vi "ADC Data capture and Process.vi"(0 "ADC Output Read Method":T2(ring)=enum."Read .dat file", 1 "Select the Tab to project":T1(ring)=enum."ADC Sine", 2 "ADC Input":enum16{"Sine Wave", "Ramp / Triangle"}(ring), 3 "No.of samples(SNR)":i32=4096, 4 "Resolution":i32=12, 5 "active edge":i32(ring)=10280, 6 "Inputs for Dyanmic para":T9={"Fundamental Frequency"=100000.0, "Sampling Frequncy"=3999610.0, "No of Harmonics"=9, "Window"=enum."7 Term B-Harris", "Blackman (fundamental power) bins)"=1.0}, 7 "Samples per Channel":i32=4096 caption="No.of Samples(capture)", 8 "Oversampling":bool, 9 "Oversampling ratio":i32, 10 "Drop LSB":bool, 11 "Save data":T15, 12 "Waveform":i64[](array[numeric]), 13 "Path to Read":path=path "C/Users/a0230227/Desktop/save.dat", 14 "Start & Stop Bit":cluster{"Start":i32, "Stop":i32}={"Start"=40, "Stop"=4055}, 15 "length":i32=4096, 24 "path to save":T14={"Path to Save plot"=path "D/Tenor_176P/DYN_PAR_C004/DAT/D001_TEMPP30C_VDD1.2_VDDA3.3_16B_SE_ADCA__vicA_aggX_PLT_CAP_200821_1740_33.jpg", "Path to Raw Data plot"=path "D/Tenor_176P/DYN_PAR_C004/DAT/D001_TEMPP30C_VDD1.2_VDDA3.3_16B_SE_ADCA__vicA_aggX_RAW_DAT_200821_1740_33.csv"}) -> (18 "Min Max":T4, 19 "detected Throughput":dbl, 20 "output cluster":T7, 21 "Dynamic Parameters":T8, 22 "max code":ext, 23 "min code":ext, 25 "Valid Capture":bool)   [LabVIEW 2021] (continued)
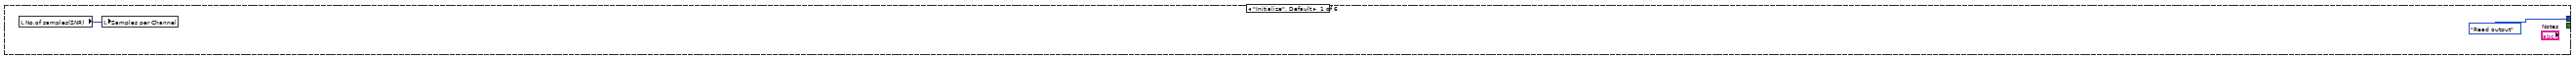
[diagram p2: hidden frame]
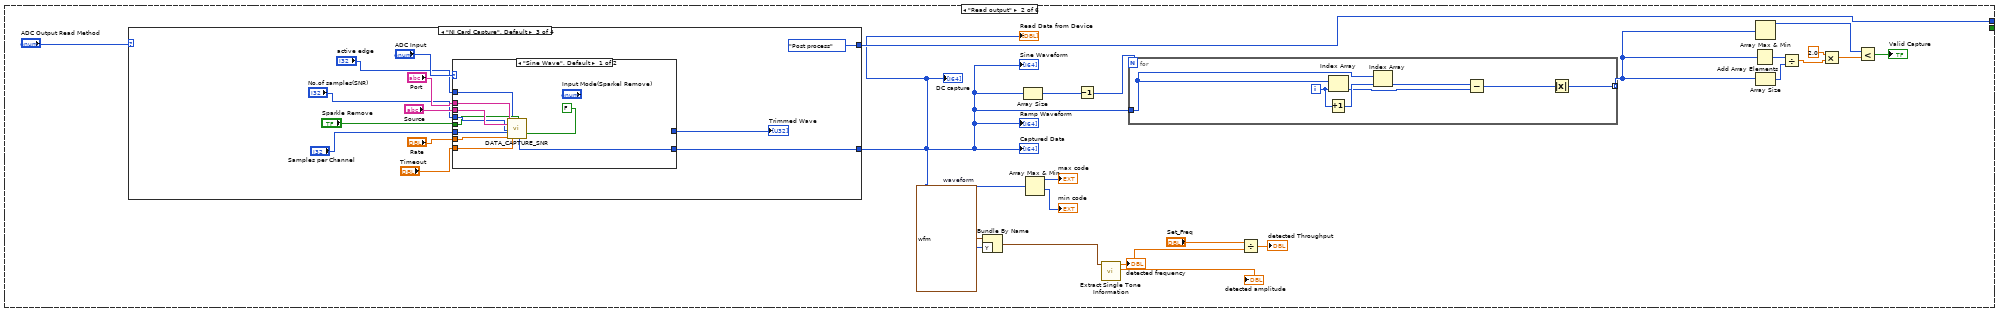
[diagram p3: hidden frame]
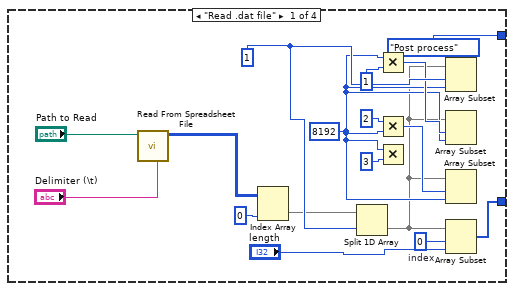
[diagram p4: hidden frame]
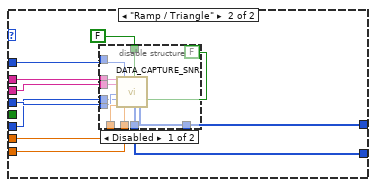
[diagram p6: hidden frame]
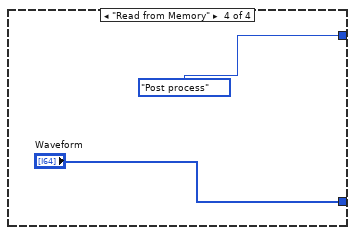
[diagram p8: hidden frame]
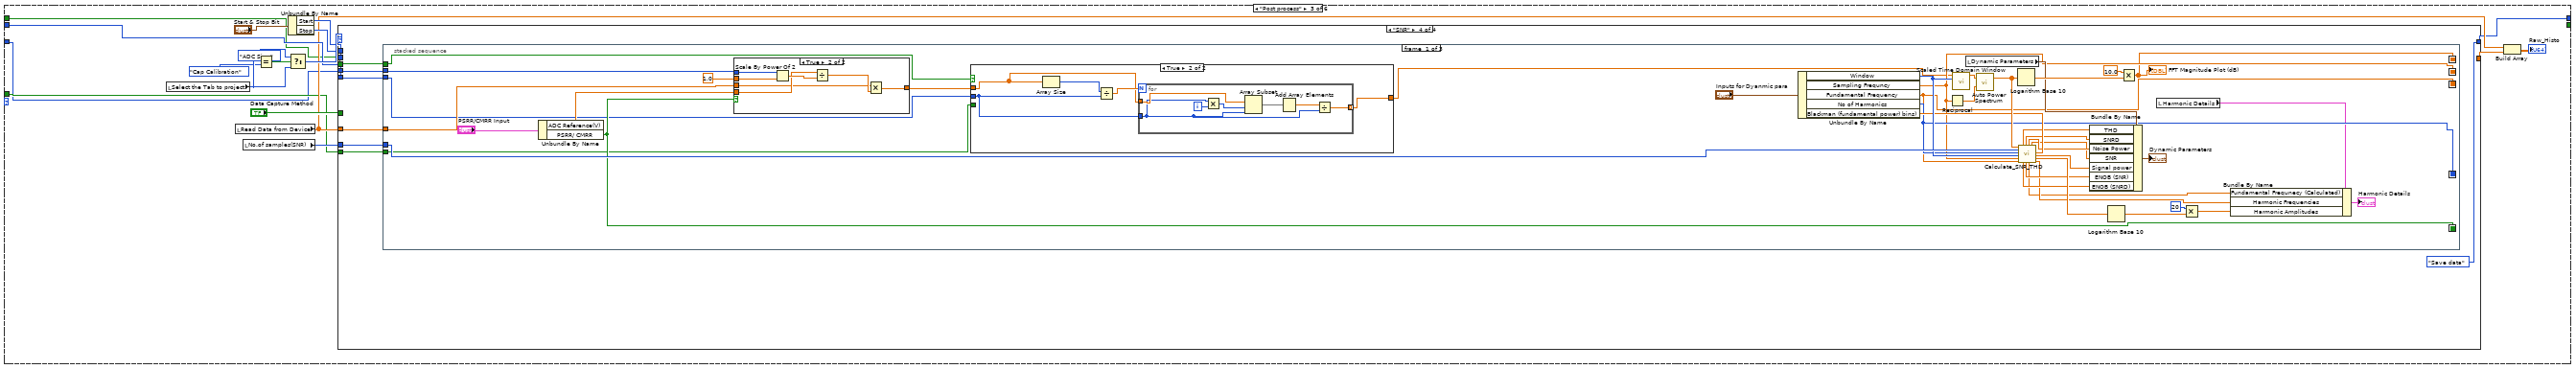
[diagram p9: hidden frame]
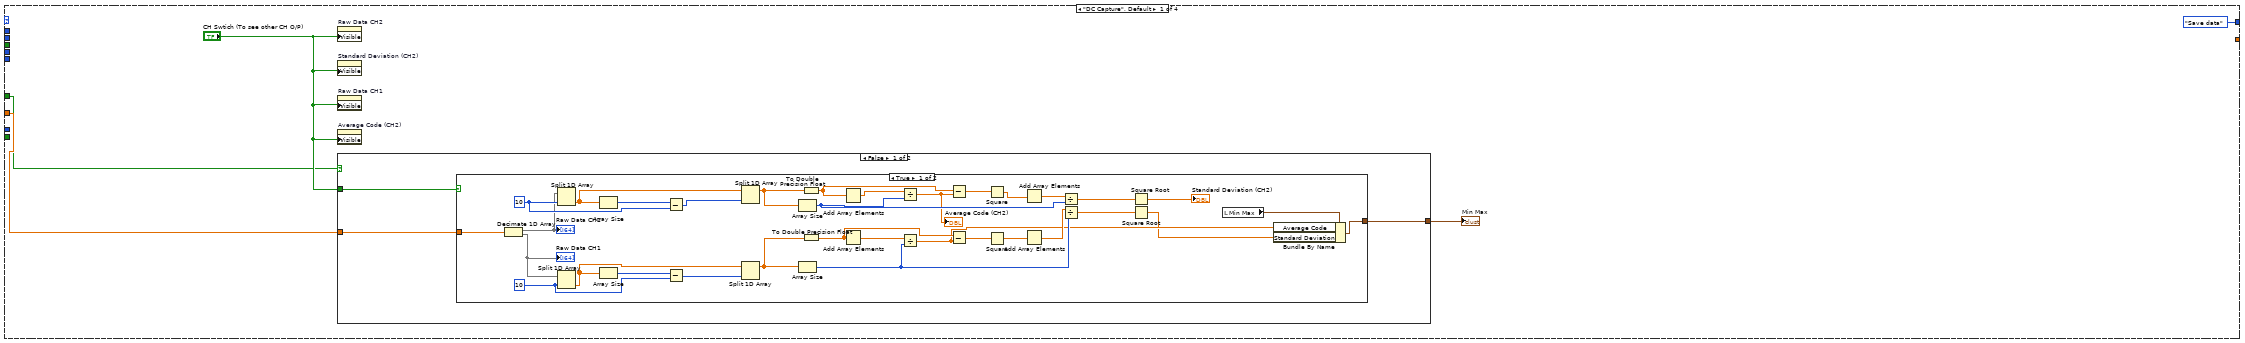
[diagram p10: hidden frame]
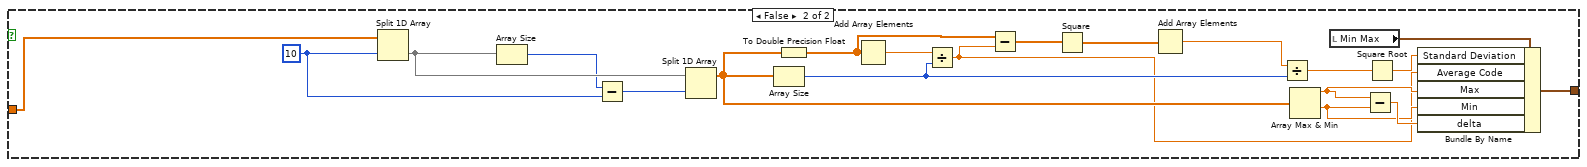
[diagram p11: hidden frame]
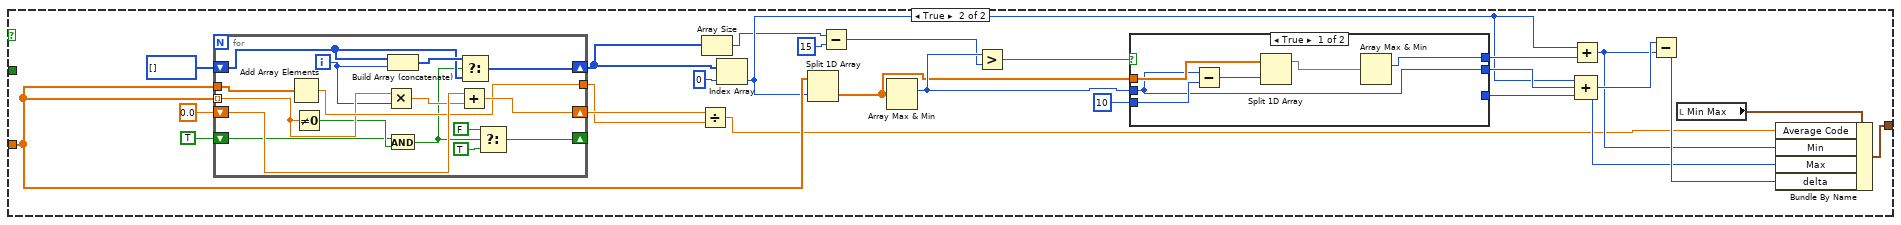
[diagram p12: hidden frame]
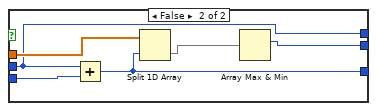
[diagram p13: hidden frame]
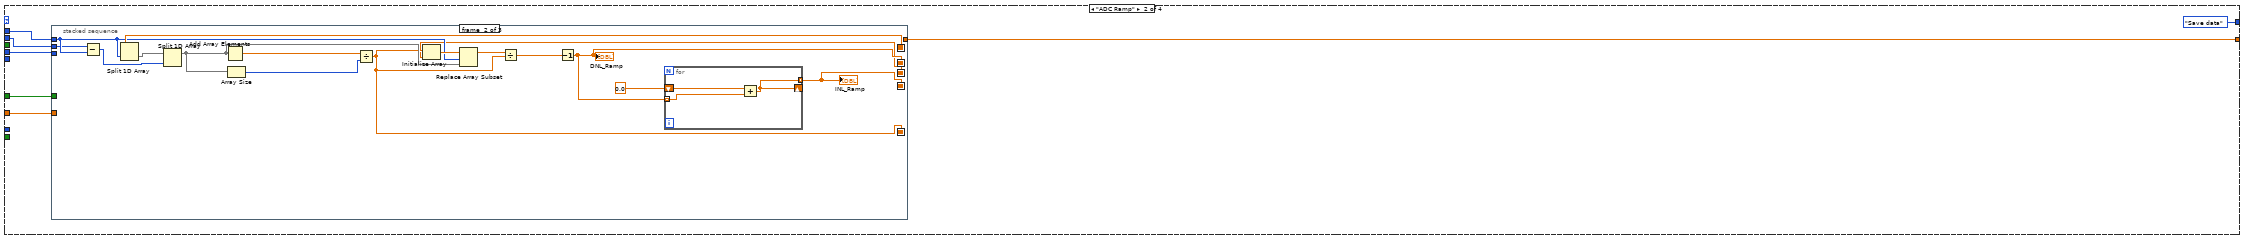
[diagram p14: hidden frame]
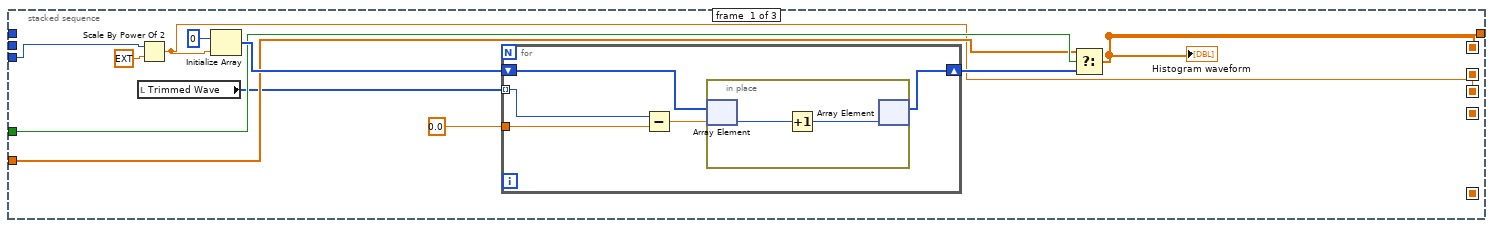
[diagram p15: hidden frame]
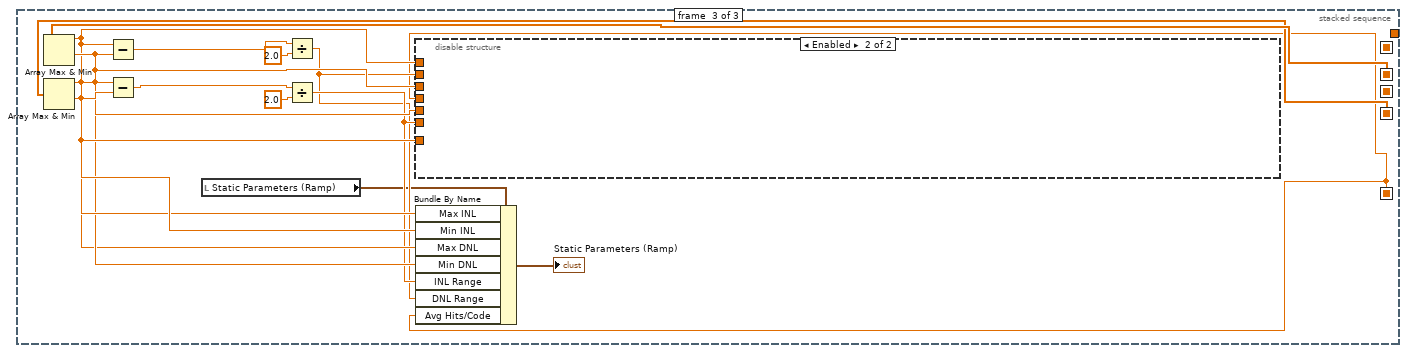
[diagram p16: hidden frame]
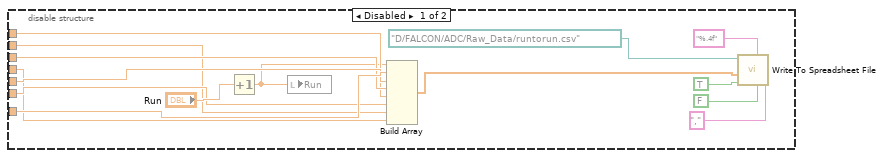
[diagram p17: hidden frame]
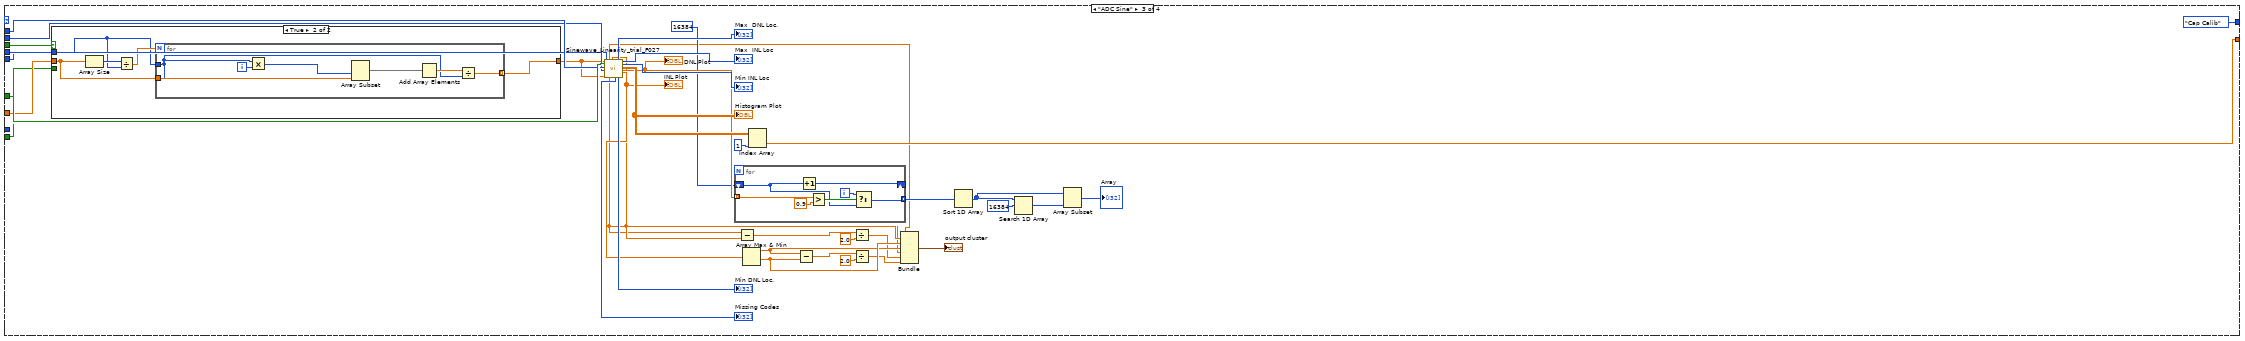
[diagram p18: hidden frame]
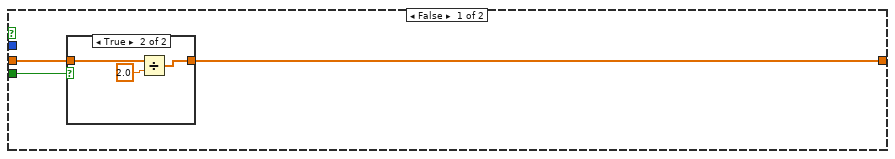
[diagram p19: hidden frame]
            n297 = case shown="True" w730 {
              tunnel: w734 -> [_ w745]
              frame False {
              }
              frame True {
                w741 = "," ("delimiter (\\t)")
                n298 = local read "Histogram Plot"() -> (w749:dbl[][])
                n299 = local read "Sine Waveform"() -> (w740:i64[])
                n300 = local read "DNL Plot"() -> (w752:dbl[])
                n301 = local read "INL Plot"() -> (w751:dbl[])
                n302 = Index Array(array=w749, index (row)=1 ("disabled index (col)")) -> (element=w748:dbl[])  [unwired: 1 in]
                n303 = call-poly <vilib>:"Write To Spreadsheet File.vi"("delimiter (\\t)"=w741, "1D data"=string[] ["DNL", "INL", "Histogram", "Rawdata"], "file path (dialog if empty)"=w745) -> ("new file path (Not A Path if cancelled)"=w744:path)  [unwired: 5 in]
                n304 = Build Array(w752, w751, w748, w740) -> (w750:dbl[][])
                n305 = call-poly <vilib>:"Write To Spreadsheet File.vi"("delimiter (\\t)"=w741, "transpose? (no:F)"=TRUE, "append to file? (new file:F)"=TRUE, "2D data"=w750, "file path (dialog if empty)"=w744) -> ()  [unwired: 3 in, 1 out]
              }
            }
            n306 = local write "Main Tab"(4) -> ()
            "Sine" <- 1
          }
          frame "SNR" {
            n307 = case shown="True" w754 {
              tunnel: w757 -> [_ w759]
              frame False {
              }
              frame True {
                n308 = Current VI's Path() -> (path=w760:path)
                n309 = call "Take fron panel screenshot.vi"("VI path"=w760, "Image path"=w759, "Visible area only? (f)"=FALSE, "File type (.jpg)"=enum16{".bmp", ".png", ".jpg"}.".png") -> ()  [unwired: 4 in, 1 out]
              }
            }
            n310 = case shown="False" w753 {
              tunnel: w756 -> [_ w765]
              frame False {
              }
              frame True {
                n311 = local read "FFT Plot"() -> (w770:cluster{dbl[], dbl[]})
                n312 = local read "Captured Data"() -> (w769:i64[])
                n313 = Unbundle(w770) -> (w768:dbl[], w767:dbl[])
                n314 = Build Array(w769, w768, w767) -> (w766:dbl[][])
                n315 = call-poly <vilib>:"Write To Spreadsheet File.vi"("delimiter (\\t)"="," ("delimiter (\\t)"), "transpose? (no:F)"=TRUE, "2D data"=w766, "file path (dialog if empty)"=w765) -> ()  [unwired: 4 in, 1 out]
              }
            }
            n316 = local write "Main Tab"(5) -> ()
            "SNR" <- 2
          }
          frame "Cap Calibration" {
            n317 = local write "Main Tab"(6) -> ()
          }
          frame "DC Capture" {
            n318 = case shown="True" w772 {
              tunnel: w773 -> [_ w778]
              frame False {
              }
              frame True {
                n319 = local read "DC capture"() -> (w775:i64[])
                n320 = call-poly <vilib>:"Write To Spreadsheet File.vi"("delimiter (\\t)"="" ("delimiter (\\t)"), "transpose? (no:F)"=TRUE, "1D data"=w775, "file path (dialog if empty)"=w778) -> ()  [unwired: 4 in, 1 out]
              }
            }
            n321 = local write "Main Tab"(2) -> ()
          }
        }
      }
      frame "Exit" {
        n322 = disable-structure shown="Enabled" {
          frame Enabled {
            w780 = FALSE ("Save INL/DNL Plot(Ramp)")
            n323 = local read "Save data"() -> (w782:T15)
            n324 = Bundle By Name(cluster=w782, "Save INL/DNL Plot(Ramp)"=w780, "Save SNR Plot"=w780, "Save INL/DNL Plot(Sine)"=w780, "Save INL/DNL Raw Data(Ramp)"=w780, "Save SNR Raw Data"=w780, "Save INL/DNL Raw Data(Sine)"=w780, "Save  Raw Data(Sine)"=w780) -> (w781:T15)
            n325 = local write "Save data"(w781) -> ()
          }
          frame Disabled {
          }
        }
        n326 = disable-structure shown="Enabled" {
          frame Disabled {
            n327 = local write item#-1(u32 12000 ("Wait time to Read Memory \n(To complete Conv) mS")) -> ()
          }
          frame Enabled {
          }
        }
      }
    }
  }
